vi "ErrorHandler.vi"(8 "Error In":errorcluster, 11 "base path":path) -> (0 "Error Out":errorcluster)   [LabVIEW 2013]
uses:
  <vilib>/Utility/error.llb/DialogType.ctl
  Controls/Error_Handler_ActionSelectTypeDef.ctl
panel:
  out "s?size max":i32
  out "size(s)":i32
  out "Array":T1(array[cluster])
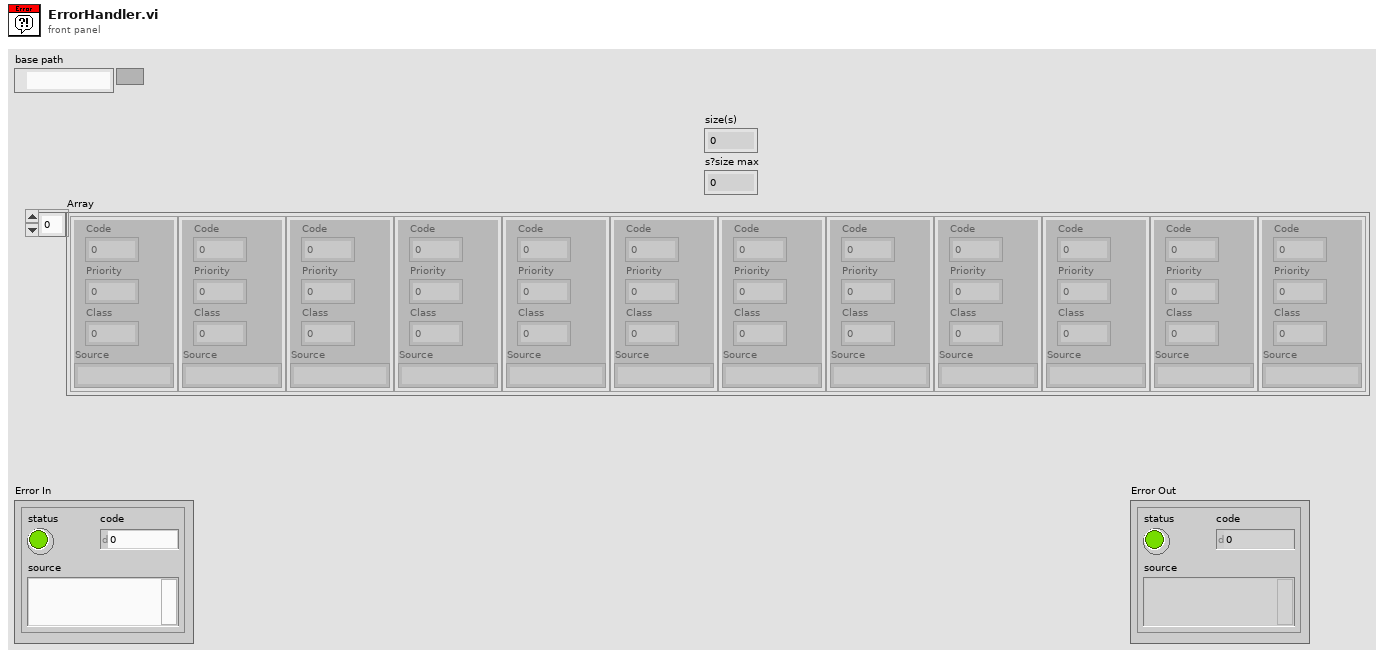
[diagram p1: front panel]
types:
  T1 = cluster{"Code":i32, "Priority":i32, "Class":i32, "Source":string}[]
  T2 = enum16{"open", "open or create", "create or replace", "create", "open (read-only)"}
  T3 = cluster{"Code":i32, "Priority":i32, "Class":i32, "Source":string}
  T4 = typedef "DialogType.ctl" = u16
  T5 = typedef "Error_Handler_ActionSelectTypeDef.ctl" = enum16{"Log", "Popup"}
  T6 = cluster{"Code":i32, "Priority":i32, "Class":i32, "string":string}
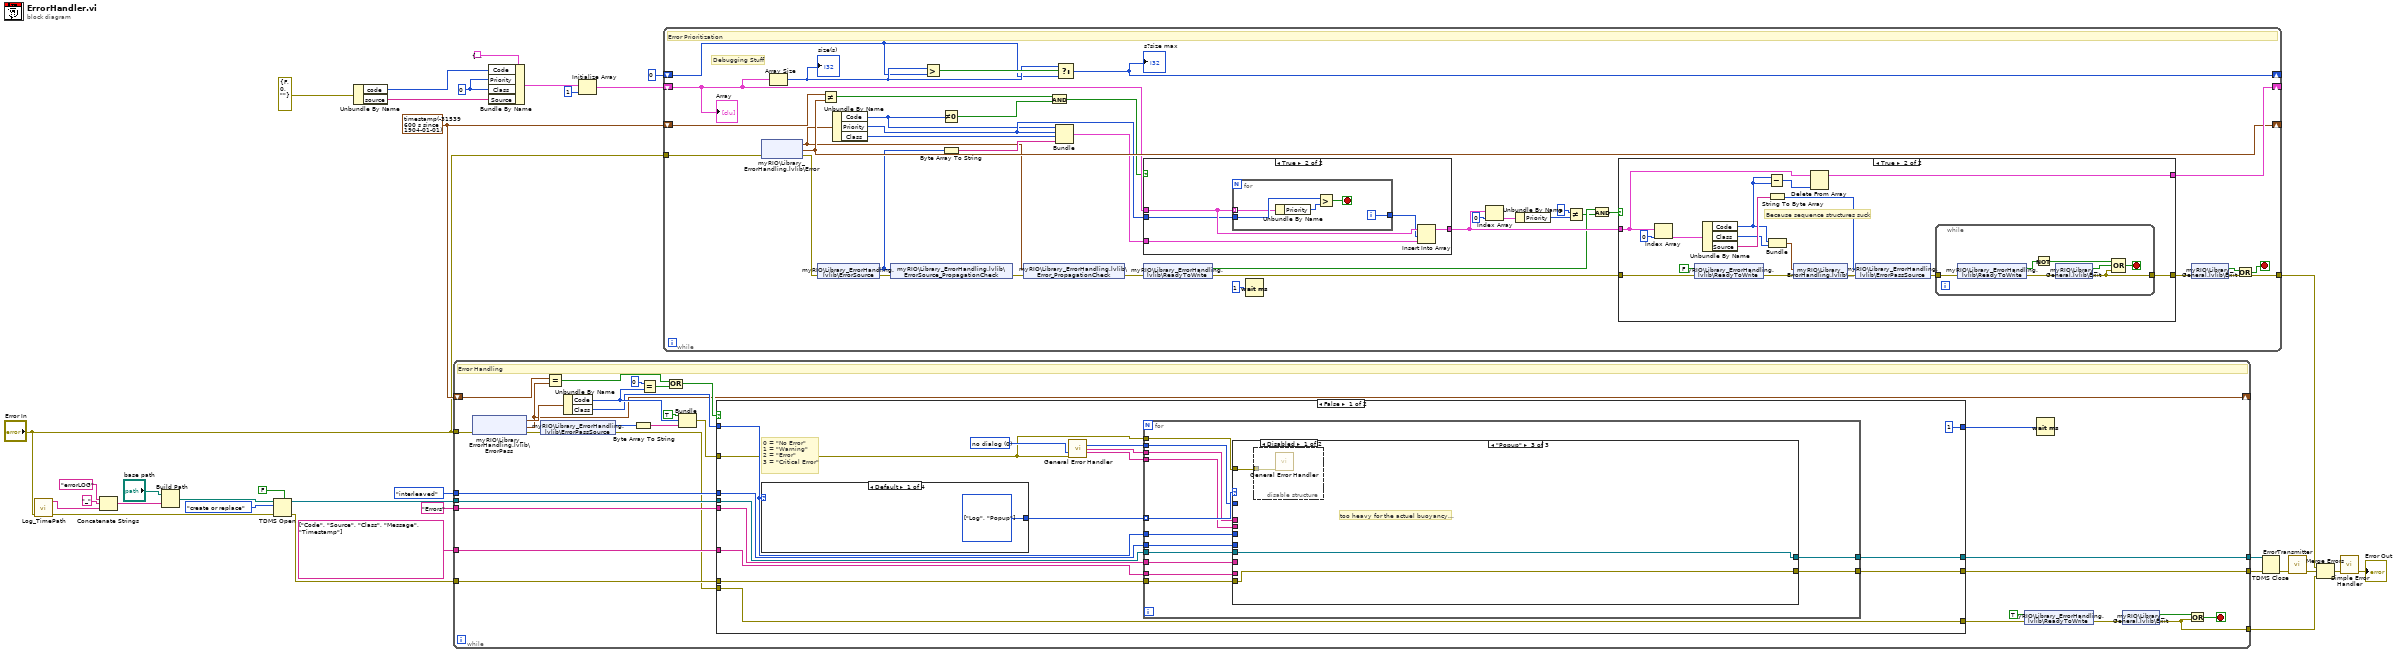
[diagram p0: block diagram]
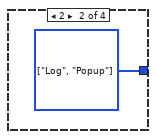
[diagram p2: hidden frame]
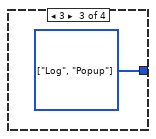
[diagram p3: hidden frame]
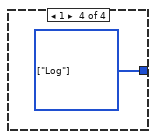
[diagram p4: hidden frame]
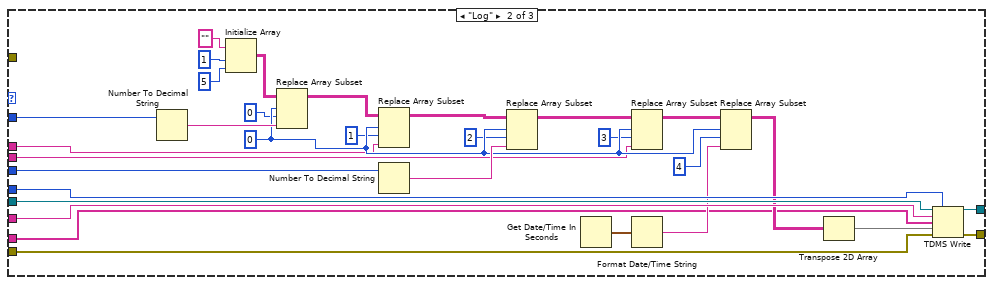
[diagram p6: hidden frame]
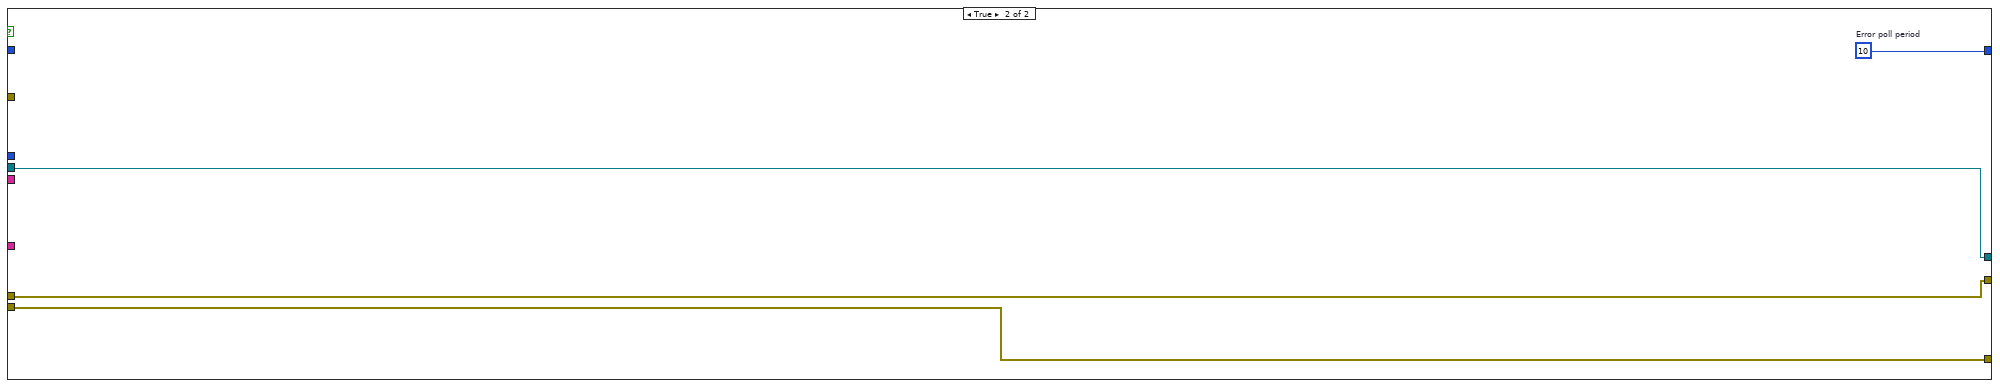
[diagram p8: hidden frame]
diagram:
  w29 = timestamp(-31539600 s since 1904-01-01)
  w30 = 0
  n1 = call "Log_TimePath.vi"("error in (no error)"="Error In") -> ("error out"=w3:errorcluster, "result string"=w22:string)  [unwired: 9 in]
  n2 = Concatenate Strings("errorLOG" ("TDMS: file name"), "_" ("string"), w22) -> (w25:string)
  n3 = Build Path(base path="base path", name or relative path=w25) -> (appended path=w21:path)
  n4 = TDMS Open(5:FALSE ("create index file? (T)"), 8:w3, 10:T2."create or replace" ("operation (0:open)"), 11:w21) -> (0:w10:errorcluster, 3:w16:refnum<k34>)  [unwired: 3 in]
  n5 = Unbundle By Name(errorcluster {"status"=FALSE, "code"=0, "source"=""} ("error constant")) -> ("code"=w32:i32, "source"=w28:string)
  n6 = while {
    shift-right: [w51] -> _
    shift-left: w29 -> [w52]
    tunnel: "Error In" -> [w49]
    tunnel: [w35] -> w12
    tunnel: enum16{"decimated", "interleaved"}."interleaved" ("data layout (0:decimated)") -> [w45]
    tunnel: "Errors" ("group name") -> [w44]
    tunnel: string[] ["Code", "Source", "Class", "Message", "Timestamp"] ("channel name(s)") -> [w43]
    tunnel: w16 -> [w42]
    tunnel: [w41] -> w15
    tunnel: w10 -> [w40]
    tunnel: [w39] -> w9
    stop <- w47 stop-if-true
    # "Error Handling"
    n7 = shared-variable "myRIO\\Library_ErrorHandling.lvlib\\ErrorPass"(error in=w49) -> (w53:cluster{"Code":i32, "Class":i32}, error out=w48:errorcluster, w51:timestamp)
    n8 = shared-variable "myRIO\\Library_ErrorHandling.lvlib\\ErrorPassSource"(error in=w48) -> (w54:u8[], error out=w37:errorcluster)
    n9 = Equal?(x=w52, y=w51) -> (x = y?=w50:bool)
    n10 = Unbundle By Name(w53) -> ("Code"=w58:i32, "Class"=w57:i32)
    n11 = Byte Array To String(unsigned byte array=w54) -> (string=w61:string)
    n12 = Equal?(x=0, y=w58) -> (x = y?=w55:bool)
    n13 = Or(x=w50, y=w55) -> (x .or. y?=w56:bool)
    n14 = Bundle(TRUE, "Code"=w58, "string"=w61) -> (w60:cluster{bool, "Code":i32, "string":string})  [unwired: 1 in]
    n15 = case shown="False" w56 {
      tunnel: [u32 1 w137] -> w63
      tunnel: w60 -> [w64 _]
      tunnel: w57 -> [w70 _]
      tunnel: w45 -> [w77 _]
      tunnel: w44 -> [w76 _]
      tunnel: w43 -> [w75 _]
      tunnel: w42 -> [w74 w135]
      tunnel: [w73 w135] -> w41
      tunnel: w40 -> [w72 w136]
      tunnel: [w71 w136] -> w39
      tunnel: w37 -> [w65 w134]
      tunnel: [w65 w134] -> w36
      frame False {
        w69 = T4 0 items=["no dialog", "OK message", "continue or stop message", "OK message + warnings", "continue/stop + warnings"] ("type of dialog (OK msg:1)")
        # "0 = \"No Error\"\n1 = \"Warning\"\n2 = \"Error\"\n3 = \"Critical Error\""
        n16 = case shown="Default" w70 {
          tunnel: [w80 w81 w82 w83] -> w78
          frame Default {
            w80 = T5[] [enum."Log", enum."Popup"] items=["Log", "Popup"] ("array 2")
          }
          frame 2 {
            w81 = T5[] [enum."Log", enum."Popup"] items=["Log", "Popup"] ("array 2")
          }
          frame 3 {
            w82 = T5[] [enum."Log", enum."Popup"] items=["Log", "Popup"] ("array 2")
          }
          frame 1 {
            w83 = T5[] [enum."Log"] items=["Log", "Popup"] ("array 2")
          }
        }
        n17 = call <vilib>:"General Error Handler.vi"("type of dialog (OK msg:1)"=w69, "error in (no error)"=w64) -> ("code out"=w66:i32, "source out"=w68:string, "message"=w67:string)  [unwired: 9 in, 2 out]
        n18 = for {
          tunnel: w78 -> [w96] mode=indexing
          tunnel: w77 -> [w95]
          tunnel: w76 -> [w94]
          tunnel: w75 -> [w93]
          tunnel: w74 -> [w92]
          tunnel: [w91] -> w73
          tunnel: w72 -> [w90]
          tunnel: [w89] -> w71
          tunnel: w70 -> [w88]
          tunnel: w68 -> [w87]
          tunnel: w67 -> [w86]
          tunnel: w66 -> [w85]
          tunnel: w64 -> [w84]
          n19 = case shown="\"Popup\"" w96 {
            tunnel: w95 -> [_ w129 _]
            tunnel: w94 -> [_ w125 _]
            tunnel: w93 -> [_ w104 _]
            tunnel: w92 -> [w97 w126 w130]
            tunnel: [w97 w128 w130] -> w91
            tunnel: w90 -> [w98 w124 w131]
            tunnel: [w98 w127 w131] -> w89
            tunnel: w88 -> [_ w123 _]
            tunnel: w87 -> [_ w101 _]
            tunnel: w86 -> [_ w100 _]
            tunnel: w85 -> [_ w99 _]
            tunnel: w84 -> [_ _ w132]
            frame Default {
            }
            frame "Log" {
              w115 = 0 ("dimension size")
              n20 = Number To Decimal String(number=w99) -> (decimal integer string=w122:string)  [unwired: 1 in]
              n21 = Initialize Array("" ("date/time string"), 1 ("dimension size"), 5 ("dimension size")) -> (w116:string[][])
              n22 = Replace Array Subset(array=w116, new element=w122, index (row)=w115, index (col)=0) -> (w110:string[][])
              n23 = Replace Array Subset(array=w110, new element=w101, index (row)=w115, index (col)=1 ("disabled index (col)")) -> (w109:string[][])
              n24 = Number To Decimal String(number=w123) -> (decimal integer string=w121:string)  [unwired: 1 in]
              n25 = Replace Array Subset(array=w109, new element=w121, index (row)=w115, index (col)=2 ("index (row)")) -> (w108:string[][])
              n26 = Get Date/Time In Seconds() -> (seconds since 1Jan1904=w120:timestamp)
              n27 = Replace Array Subset(array=w108, new element=w100, index (row)=w115, index (col)=3 ("disabled index (col)")) -> (w107:string[][])
              n28 = Format Date/Time String(seconds (now)=w120) -> (date/time string=w119:string)  [unwired: 2 in]
              n29 = Replace Array Subset(array=w107, new element=w119, index (row)=w115, index (col)=4 ("index (row)")) -> (w106:string[][])
              n30 = Transpose 2D Array(2D array=w106) -> (transposed array=w105:string[][])
              n31 = TDMS Write(0:w126, 1:w129, 5:w125, 7:w104, 9:w105, 11:w124) -> (4:w128:refnum<k34>, 15:w127:errorcluster)  [unwired: 2 out]
            }
            frame "Popup" {
              # "too heavy for the actuel buoyancy..."
              n32 = disable-structure shown="Disabled" {
                disable-tunnel: w132 -> [w133 _]
                frame Disabled {
                  n33 = call <vilib>:"General Error Handler.vi"("error in (no error)"=w133) -> ()  [unwired: 10 in, 5 out]
                }
                frame Enabled {
                }
              }
            }
          }
        }
      }
      frame True {
        w137 = u32 10  # Error poll period
      }
    }
    n34 = shared-variable "myRIO\\Library_ErrorHandling.lvlib\\ReadyToWrite"(TRUE, error in=w36) -> (error out=w34:errorcluster)
    n35 = Wait (ms)(milliseconds to wait=w63) -> ()  [unwired: 1 out]
    n36 = shared-variable "myRIO\\Library_General.lvlib\\Exit"(error in=w34) -> (w46:bool, error out=w35:errorcluster)
    n37 = Or(x=w46, y=w35) -> (x .or. y?=w47:bool)
  }
  n38 = Bundle By Name(cluster=T3 {"Code"=0, "Priority"=0, "Class"=0, "Source"=""} ("Error"), "Code"=w32, "Priority"=w30, "Class"=w30, "Source"=w28) -> (w31:T3)
  n39 = Initialize Array(w31, 1 ("dimension size")) -> (w1:T1)
  n40 = while {
    shift-right: [w174] -> _
    shift-left: w1 -> [w144]
    shift-right: [w161] -> _
    shift-left: w29 -> [w165]
    tunnel: "Error In" -> [w160]
    tunnel: [w138] -> w5
    shift-right: [w145] -> _
    shift-left: 0 ("y") -> [w146]
    stop <- w162 stop-if-true
    # "Debugging Stuff"
    # "Error Prioritization"
    n41 = shared-variable "myRIO\\Library_ErrorHandling.lvlib\\Error"(error in=w160) -> (w150:cluster{"Code":i32, "Priority":i32, "Class":i32}, error out=w159:errorcluster, w161:timestamp)
    n42 = Array Size(array=w144) -> (size(s)=w147:i32)
    "size(s)" <- w147
    n43 = shared-variable "myRIO\\Library_ErrorHandling.lvlib\\ErrorSource"(error in=w159) -> (w149:u8[], error out=w153:errorcluster)
    n44 = Not Equal?(x=w165, y=w161) -> (x != y?=w141:bool)
    n45 = Unbundle By Name(w150) -> ("Code"=w143:i32, "Priority"=w157:i32, "Class"=w156:i32)
    n46 = shared-variable "myRIO\\Library_ErrorHandling.lvlib\\ErrorSource_PropagationCheck"(w149, error in=w153) -> (error out=w152:errorcluster)
    n47 = Greater?(x=w147, y=w146) -> (0:w148:bool)
    n48 = Not Equal To 0?(x=w143) -> (x != 0?=w142:bool)
    n49 = Byte Array To String(unsigned byte array=w149) -> (string=w155:string)
    n50 = shared-variable "myRIO\\Library_ErrorHandling.lvlib\\Error_PropagationCheck"(w150, error in=w152) -> (error out=w151:errorcluster)
    n51 = And(x=w141, y=w142) -> (x .and. y?=w140:bool)
    n52 = Bundle("Code"=w143, "Priority"=w157, "Class"=w156, "string"=w155) -> (w158:T6)  [unwired: 1 in]
    n53 = Select(t=w147, s=w148, f=w146) -> (s? t:f=w145:i32)
    "s?size max" <- w145
    n54 = case shown="True" w140 {
      tunnel: w144 -> [w175 w180]
      tunnel: w157 -> [_ w179]
      tunnel: w158 -> [_ w176]
      tunnel: [w175 w177] -> w173
      frame False {
      }
      frame True {
        n55 = for {
          tunnel: w179 -> [w185]
          tunnel: [w181] -> w178
          tunnel: w180 -> [w183] mode=indexing
          i -> [w181]
          stop <- w184 stop-if-true
          n56 = Unbundle By Name(w183) -> ("Priority"=w182:i32)
          n57 = Greater?(x=w185, y=w182) -> (0:w184:bool)
        }
        n58 = Insert Into Array(array=w180, index=w178, new element=w176) -> (w177:T1)
      }
    }
    n59 = shared-variable "myRIO\\Library_ErrorHandling.lvlib\\ReadyToWrite"(error in=w151) -> (w170:bool, error out=w164:errorcluster)
    n60 = Wait (ms)(milliseconds to wait=u32 1) -> ()  [unwired: 1 out]
    n61 = Index Array(array=w173, index=0) -> (element=w167:T3)
    n62 = Unbundle By Name(w167) -> ("Priority"=w166:i32)
    n63 = Not Equal?(x=0, y=w166) -> (x != y?=w168:bool)
    n64 = And(x=w170, y=w168) -> (x .and. y?=w169:bool)
    n65 = case shown="True" w169 {
      tunnel: w173 -> [w187 w193]
      tunnel: [w187 w202] -> w174
      tunnel: [w186 w188] -> w139
      tunnel: w164 -> [w186 w194]
      frame False {
      }
      frame True {
        # "Because sequence structures suck"
        n66 = Index Array(array=w193, index=0) -> (element=w201:T3)
        n67 = shared-variable "myRIO\\Library_ErrorHandling.lvlib\\ReadyToWrite"(FALSE, error in=w194) -> (error out=w195:errorcluster)
        n68 = Unbundle By Name(w201) -> ("Code"=w192:i32, "Class"=w199:i32, "Source"=w200:string)
        n69 = Subtract(x=w192, y=w192) -> (x-y=w190:i32)
        n70 = String To Byte Array(string=w200) -> (unsigned byte array=w197:u8[])
        n71 = Bundle("Code"=w192, "Class"=w199) -> (w198:cluster{"Code":i32, "Class":i32})  [unwired: 1 in]
        n72 = shared-variable "myRIO\\Library_ErrorHandling.lvlib\\ErrorPass"(w198, error in=w195) -> (error out=w196:errorcluster)
        n73 = Delete From Array(array=w193, index=w190) -> (array with subset deleted=w202:T1)  [unwired: 1 in, 1 out]
        n74 = shared-variable "myRIO\\Library_ErrorHandling.lvlib\\ErrorPassSource"(w197, error in=w196) -> (error out=w189:errorcluster)
        n75 = while {
          tunnel: w189 -> [w209]
          tunnel: [w204] -> w188
          stop <- w206 stop-if-true
          n76 = shared-variable "myRIO\\Library_ErrorHandling.lvlib\\ReadyToWrite"(error in=w209) -> (w210:bool, error out=w205:errorcluster)
          n77 = Not(x=w210) -> (.not. x?=w208:bool)
          n78 = shared-variable "myRIO\\Library_General.lvlib\\Exit"(error in=w205) -> (w207:bool, error out=w204:errorcluster)
          n79 = Compound Arithmetic op=OR(w208, w207, w204) -> (w206:bool)
        }
      }
    }
    n80 = shared-variable "myRIO\\Library_General.lvlib\\Exit"(error in=w139) -> (w163:bool, error out=w138:errorcluster)
    n81 = Or(x=w163, y=w138) -> (x .or. y?=w162:bool)
    "Array" <- w144
  }
  n82 = TDMS Close(8:w9, 11:w15) -> (0:w14:errorcluster)  [unwired: 1 out]
  n83 = call "ErrorTransmitter.vi"("Error In"=w14) -> ("Error Out"=w11:errorcluster)  [unwired: 10 in]
  n84 = Merge Errors(w5, w11, w12) -> (w13:errorcluster)
  n85 = call <vilib>:"Simple Error Handler.vi"("error in (no error)"=w13) -> ("error out"=→"Error Out":errorcluster)  [unwired: 4 in, 4 out]
